vi "MagPS_time_interlock.vi"(6 "time_in":i32 caption="Time Elapsed", 8 "time_max":i32=600 caption="Max Time", 9 "unusual_cont_lock":refnum<vi>, 10 "all_cont_lock":refnum<vi>, 11 "enable_time_limit":bool caption="Time Limit") -> (1 "status_time":u32(colorbox)=9567230, 4 "time_out":i32 caption="Time Elapsed")   [LabVIEW 2019]
doc: "This example demonstrates how to simulate a general PID controller."
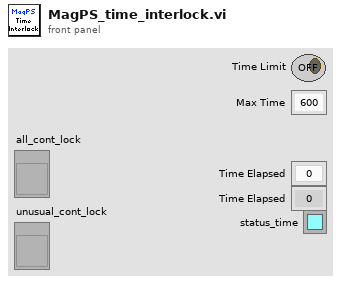
[diagram p1: front panel]
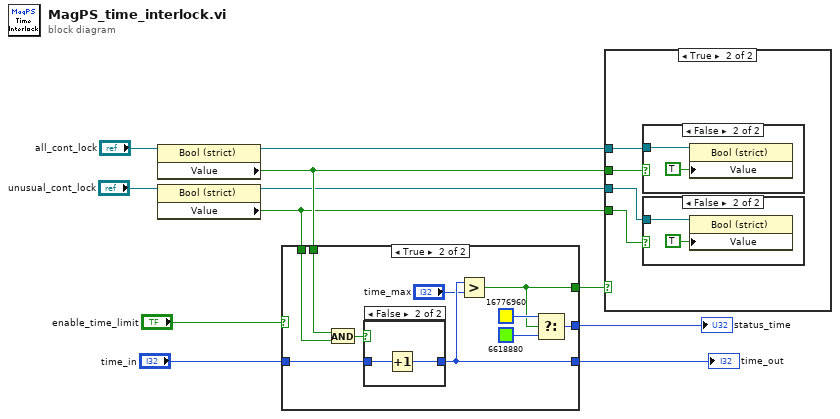
[diagram p0: block diagram]
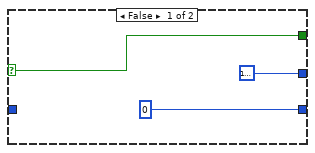
[diagram p2: hidden frame]
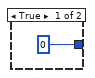
[diagram p3: hidden frame]
diagram:
  n1 = property class="Bool (strict)"(reference="all_cont_lock") -> (reference out=w9:refnum<vi>, "Value"=w4:bool)  [unwired: 1 in, 1 out]
  n2 = property class="Bool (strict)"(reference="unusual_cont_lock") -> (reference out=w1:refnum<vi>, "Value"=w2:bool)  [unwired: 1 in, 1 out]
  n3 = case shown="True" "enable_time_limit" {
    selector: "enable_time_limit" -> [w14 _]
    tunnel: "time_in" -> [_ w24]
    tunnel: [0 w23] -> w10
    tunnel: w4 -> [_ w16]
    tunnel: [w14 w18] -> w8
    tunnel: [u32 16777222 ("alarm_status") w19] -> w6
    tunnel: w2 -> [_ w15]
    frame False {
    }
    frame True {
      n4 = And(x=w16, y=w15) -> (x .and. y?=w17:bool)
      n5 = case shown="False" w17 {
        tunnel: w24 -> [_ w27]
        tunnel: [0 w26] -> w23
        frame True {
        }
        frame False {
          n6 = Increment(x=w27) -> (x+1=w26:i32)
        }
      }
      n7 = Greater?(x=w23, y="time_max") -> (0:w18:bool)
      n8 = Select(t=u32 16776960 ("alarm_status"), s=w18, f=u32 6618880 ("alarm_status")) -> (s? t:f=w19:u32)
    }
  }
  "time_out" <- w10
  "status_time" <- w6
  n9 = case shown="True" w8 {
    tunnel: w9 -> [_ w31]
    tunnel: w4 -> [_ w30]
    tunnel: w2 -> [_ w29]
    tunnel: w1 -> [_ w28]
    frame False {
    }
    frame True {
      n10 = case shown="False" w30 {
        tunnel: w31 -> [_ w35]
        frame True {
        }
        frame False {
          n11 = property class="Bool (strict)"(reference=w35, "Value"=TRUE) -> ()  [unwired: 1 in, 2 out]
        }
      }
      n12 = case shown="False" w29 {
        tunnel: w28 -> [_ w33]
        frame True {
        }
        frame False {
          n13 = property class="Bool (strict)"(reference=w33, "Value"=TRUE) -> ()  [unwired: 1 in, 2 out]
        }
      }
    }
  }
